vi "Register Worker with Dispatcher.vi"(8 "error in (no error)":errorcluster, 11 "Worker In":refnum<class "Worker.lvclass">) -> (0 "error out":errorcluster, 3 "Worker Out":refnum<class "Worker.lvclass">)   [LabVIEW 2020, in "Worker.lvclass"]
uses:
  Worker.lvclass
  C:/Users/anton/Documents/GitHub/Triarc-Examples/Coffee Shop/Process Job/Job Handler.lvclass
  Worker.lvclass/Worker.ctl
  Process Job/Job Handler.lvclass
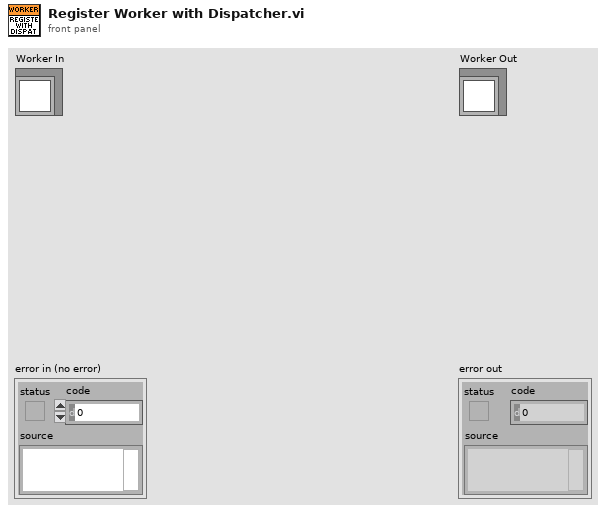
[diagram p1: front panel]
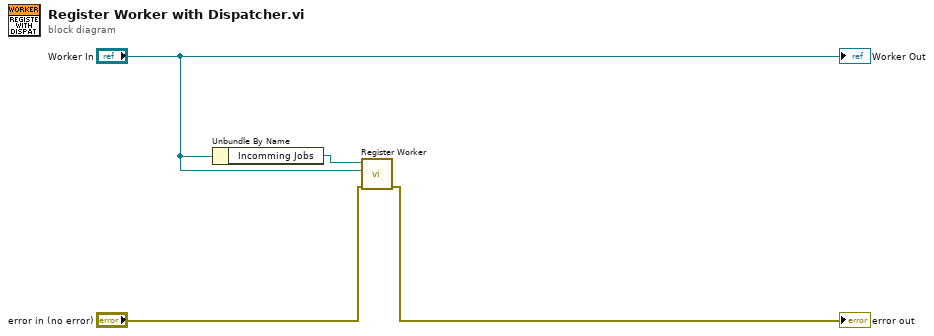
[diagram p0: block diagram]
diagram:
  n1 = Unbundle By Name("Worker In") -> ("Incomming Jobs"=w4:refnum<class "Job Handler.lvclass">)
  n2 = call-dynamic "Register Worker.vi"("error in (no error)"="error in (no error)", "Worker"="Worker In", "Job Handler In"=w4) -> ("error out"=→"error out":errorcluster)  [unwired: 7 in, 1 out]
  "Worker Out" <- "Worker In"
